vi "Initialize Front Panel.vi"(8 "error in (no error)":errorcluster, 11 "For Loop Dialog in":refnum<class "Name Only Dialog.lvclass">) -> (0 "error out":errorcluster, 3 "For Loop Dialog out":refnum<class "Name Only Dialog.lvclass">)   [LabVIEW 2017, in "Name Only Dialog.lvclass"]
doc: "<License>\nCopyright © 2017 Composed Systems, LLC | All rights reserved\nwww.composed.io\n\nAuthor: Ethan Stern <ethan.stern@composed.io>\n\nThis software is provided \"AS IS\" WITHOUT WARRANTIES, either express or implied, AND IS FOR EDUCATIONAL PURPOSES ONLY.\n</License>"
uses:
  <vilib>/gpm_packages/@cs/Test-executive-builder/Source/Test Executive Builder Dialogs/Name Only Dialog/Name Only Dialog.lvclass
  <vilib>/gpm_packages/@cs/Test-executive-builder/Source/Test Executive Builder Dialogs/Name Only Dialog/Name Only Dialog.lvclass/Name Only Dialog.ctl
  <vilib>/gpm_packages/@cs/Test-executive-builder/Source/Test Executive Builder Dialogs/ITest Executive Builder Dialog/ITest Executive Builder Dialog.lvclass
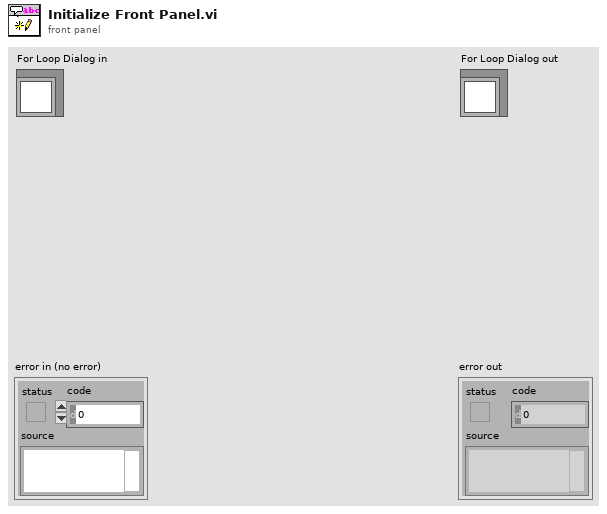
[diagram p1: front panel]
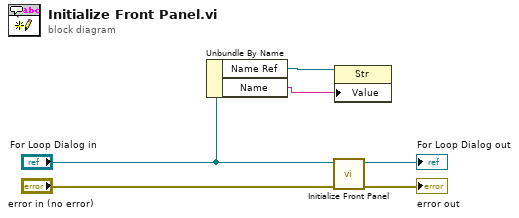
[diagram p0: block diagram]
diagram:
  n1 = Unbundle By Name("For Loop Dialog in") -> ("Name Ref"=w2:refnum<vi>, "Name"=w1:string)
  n2 = call-parent "Initialize Front Panel.vi"("error in (no error)"="error in (no error)", "ITest Executive Builder Dialog in"="For Loop Dialog in") -> ("error out"=→"error out":errorcluster, "ITest Executive Builder Dialog out"=→"For Loop Dialog out":refnum<class "Name Only Dialog.lvclass">)  [unwired: 8 in]
  n3 = property class="Str"(reference=w2, "Value"=w1) -> ()  [unwired: 1 in, 2 out]
